vi "Append_waveform_to_disk_Dlog.vi"(0 "Waveform_main":waveform(sgl), 5 "Total_samples":i32, 7 "Total_Records":i32, 9 "File#":u8) -> (15 "error out":errorcluster)   [LabVIEW 2017]
uses:
  <vilib>/Waveform/WDTFileIO.llb/ Write Waveform to File.vi
panel:
  out "JSON string":string
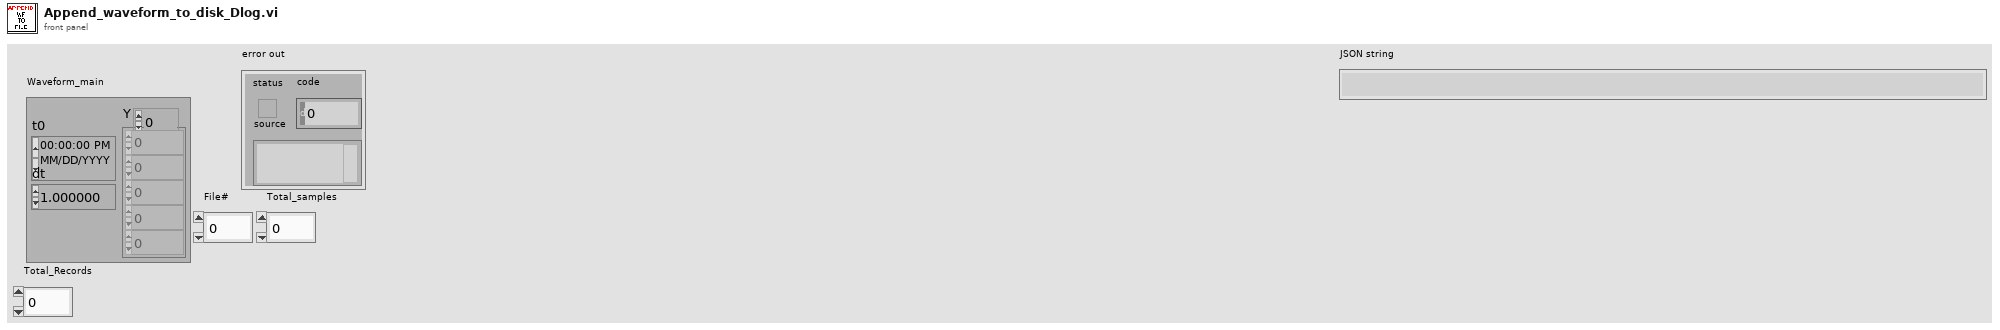
[diagram p1: front panel]
types:
  T1 = enum16{"open", "replace", "create", "open or create", "replace or create", "replace or create with confirmation"}
  T2 = cluster{"File#":u8, "Total_samples":i32, "Total_Records":i32}
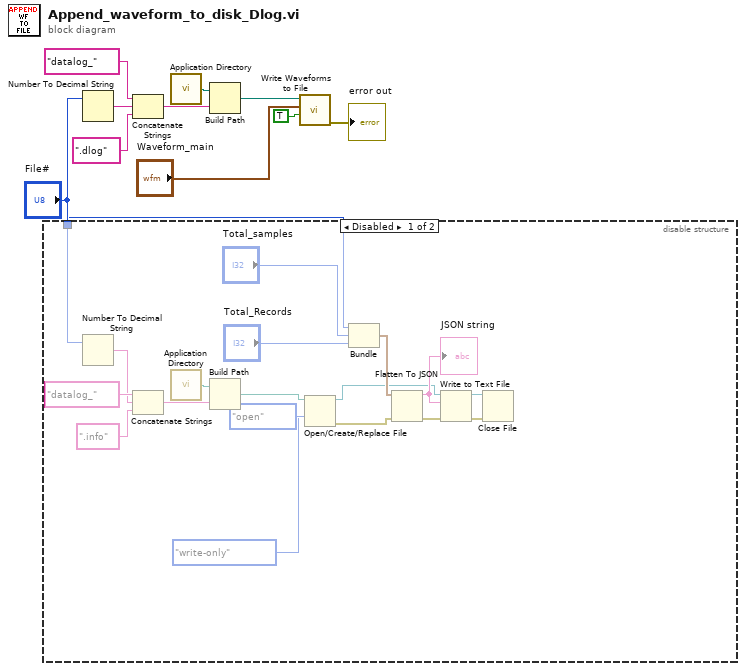
[diagram p0: block diagram]
diagram:
  n1 = disable-structure shown="Disabled" {
    disable-tunnel: "File#" -> [w20 _]
    frame Disabled {
      n2 = Number To Decimal String(number=w20) -> (decimal integer string=w27:string)  [unwired: 1 in]
      n3 = Concatenate Strings("datalog_" ("string"), w27, ".info" ("string")) -> (w24:string)
      n4 = call <vilib>:"Application Directory.vi"() -> ("Application Directory"=w25:path)
      n5 = Build Path(base path=w25, name or relative path=w24) -> (appended path=w15:path)
      n6 = Open/Create/Replace File(file path (use dialog)=w15, operation (0:open)=T1."open", access (0:read/write)=enum16{"read/write", "read-only", "write-only"}."write-only") -> (refnum out=w13:refnum<file>, error out=w12:errorcluster)  [unwired: 3 in, 1 out]
      n7 = Bundle("File#"=w20, "Total_samples"="Total_samples", "Total_Records"="Total_Records") -> (w21:T2)  [unwired: 1 in]
      n8 = Flatten To JSON(anything=w21, error in (no error)=w12) -> (JSON string=w18:string, 11:w19:errorcluster)  [unwired: 1 in]
      "JSON string" <- w18
      n9 = Write to Text File(file (use dialog)=w13, text=w18, error in=w19) -> (refnum out=w17:refnum<file>, error out=w16:errorcluster)  [unwired: 1 in, 1 out]
      n10 = Close File(refnum=w17, error in=w16) -> ()  [unwired: 2 out]
    }
    frame Enabled {
    }
  }
  n11 = Number To Decimal String(number="File#") -> (decimal integer string=w3:string)  [unwired: 1 in]
  n12 = Concatenate Strings("datalog_" ("string"), w3, ".dlog" ("string")) -> (w2:string)
  n13 = call <vilib>:"Application Directory.vi"() -> ("Application Directory"=w10:path)
  n14 = Build Path(base path=w10, name or relative path=w2) -> (appended path=w7:path)
  n15 = call-poly <vilib>:"Write Waveforms to File.vi"("append to file? (new file:F)"=TRUE, "waveform"="Waveform_main", "file path (dialog if empty)"=w7) -> ("error out"=→"error out":errorcluster)  [unwired: 7 in, 1 out]
